vi "Create.vi"(8 "error in (no error)":errorcluster) -> (0 "error out":errorcluster, 3 "Identical Comparator":refnum<class "Identical Comparator.lvclass">)   [LabVIEW 2020, in "Identical Comparator.lvclass"]
uses:
  Identical Comparator.lvclass
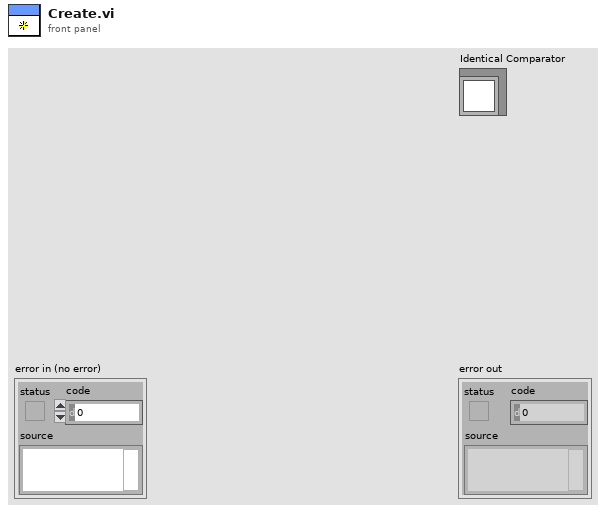
[diagram p1: front panel]
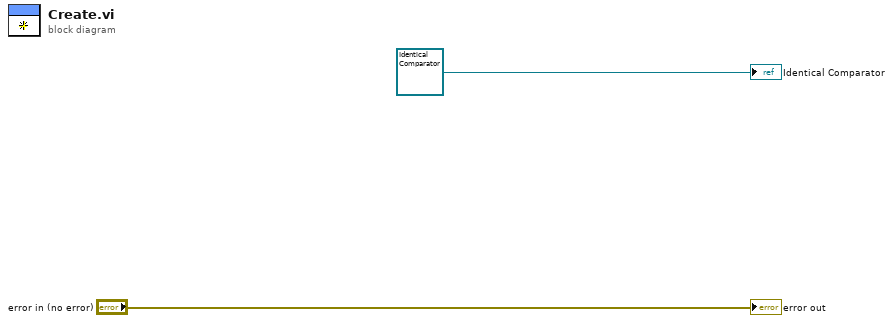
[diagram p0: block diagram]
diagram:
  "error out" <- "error in (no error)"
  "Identical Comparator" <- refnum<class "Identical Comparator.lvclass"> refnum ("Identical Comparator")
